vi "ABB configure Report.vi"() -> ()   [LabVIEW 2017]
uses:
  ABB global.vi
panel:
  in  "Select":bool
  in  "Report Templates":u16(ring) items=["testreport 11082020.html", "testreport.html", "testreport6.html"]
  out "Selected Report template":string
  in  "Exit":bool
  # "Configure Report"
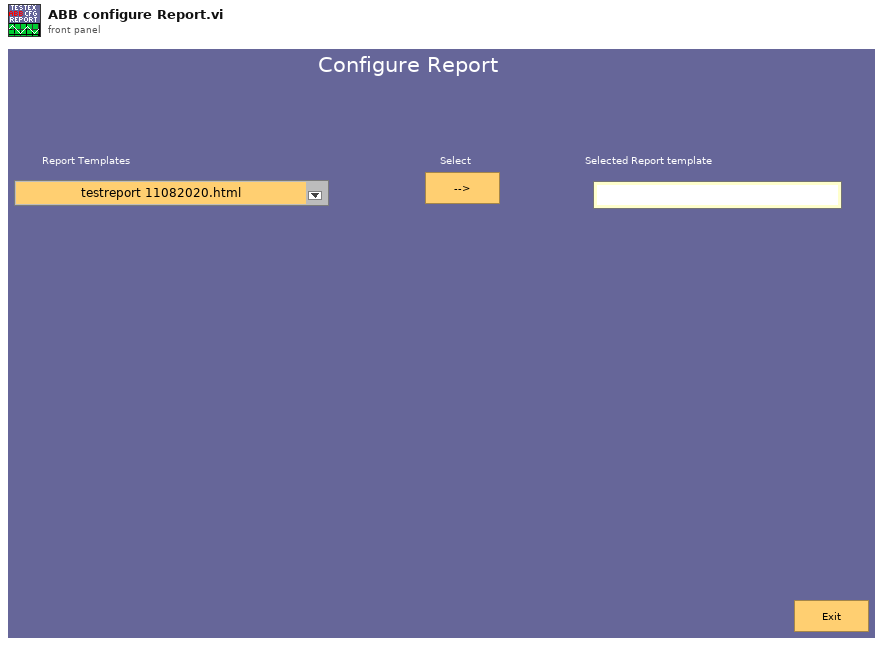
[diagram p1: front panel]
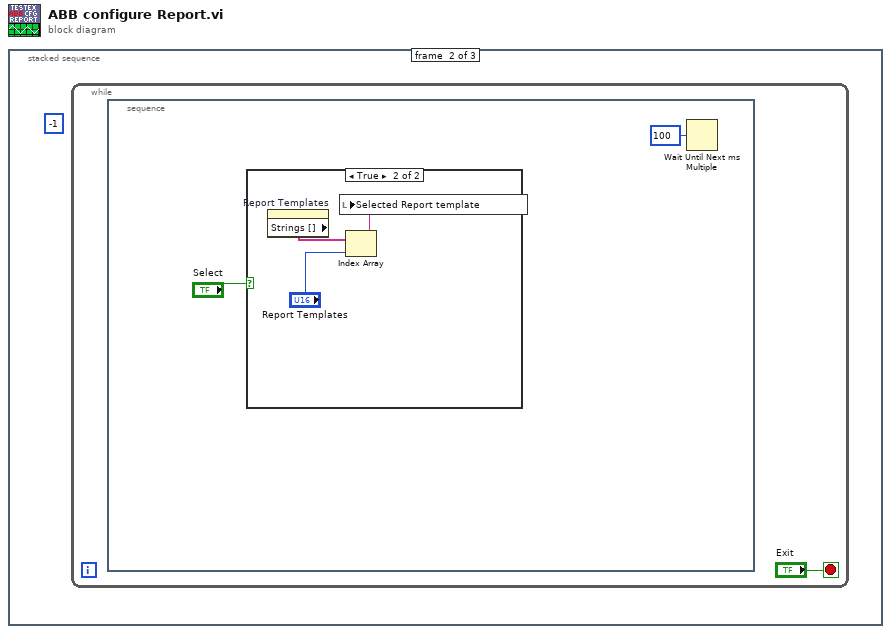
[diagram p0: block diagram]
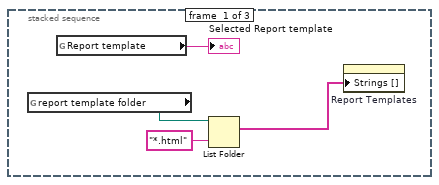
[diagram p2: hidden frame]
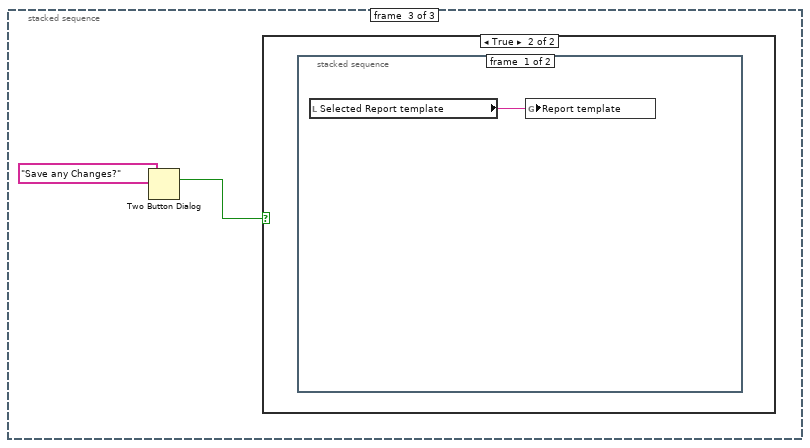
[diagram p4: hidden frame]
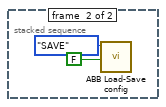
[diagram p6: hidden frame]
diagram:
  n1 = stacked-sequence {
    frame #0 {
      n2 = global read "ABB global.vi" "report template folder"() -> (w3:path)
      n3 = global read "ABB global.vi" "Report template"() -> (→"Selected Report template":string)
      n4 = List Folder(path=w3, pattern="*.html") -> (filenames=w1:string[])  [unwired: 2 in, 3 out]
      n5 = property on="Report Templates" class="Ring (strict)"("Strings []"=w1) -> ()  [unwired: 2 in, 2 out]
    }
    frame #1 {
      (unwired) -1 ("Number Values")
      n6 = while {
        stop <- "Exit" stop-if-true
        n7 = stacked-sequence {
          frame #0 {
            n8 = case shown="True" "Select" {
              frame False {
              }
              frame True {
                n9 = property on="Report Templates" class="Ring (strict)"() -> ("Strings []"=w10:string[])  [unwired: 2 in, 2 out]
                n10 = Index Array(array=w10, index="Report Templates") -> (element=w9:string)
                n11 = local write "Selected Report template"(w9) -> ()
              }
            }
            n12 = Wait Until Next ms Multiple(millisecond multiple=u32 100) -> ()  [unwired: 1 out]
          }
        }
      }
    }
    frame #2 {
      n13 = Two Button Dialog(message="Save any Changes?") -> (T button?=w12:bool)  [unwired: 2 in]
      n14 = case shown="True" w12 {
        frame False {
        }
        frame True {
          n15 = stacked-sequence {
            frame #0 {
              n16 = local read "Selected Report template"() -> (w13:string)
              n17 = global write "ABB global.vi" "Report template"(w13) -> ()
            }
            frame #1 {
              n18 = call "ABB Load-Save config.vi"("confirm save"=FALSE, "Mode"=enum16{"LOAD", "SAVE"}."SAVE") -> ()  [unwired: 10 in]
            }
          }
        }
      }
    }
  }
